vi "file read and write.vi"() -> (2 "data match?":bool)   [LabVIEW 2013, in "Shared Memory Tests.lvlib"]
uses:
  Shared Memory Tests.lvlib
  module/execution/Shared Memory Runtime.lvclass
  module/configuration/Shared Memory Configuration.lvclass
  <vilib>/NI/Tag Bus/dictionary/data dictionary.lvclass/data dictionary.ctl
  <vilib>/Analysis/1siggen.llb/Ramp Pattern by Samples.vi
  <vilib>/NI/Tag Bus/dictionary/lookup polymorphs/locate double.vi
  <vilib>/NI/Tag Bus/table/data polymorphs/write many/write Doubles.vi
  <vilib>/NI/Tag Bus/table/data polymorphs/read many/read Doubles.vi
  <vilib>/NI/Tag Bus/dictionary/search/find data index.vi
  <vilib>/NI/Tag Bus/dictionary/search/search string list.vi
  <vilib>/NI/Tag Bus/dictionary/tag not found.vi
  <vilib>/Analysis/NI_AALBase.lvlib
  <vilib>/NI/Tag Bus/table/data table.lvlib
  <vilib>/NI/Tag Bus/dictionary/data dictionary.lvclass
panel:
  out "error out":errorcluster
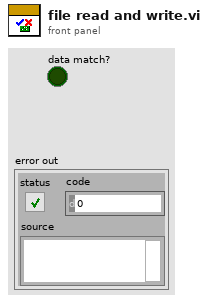
[diagram p1: front panel]
types:
  T1 = typedef "TBM channel.lvclass/data tables.ctl" = cluster{"input data":T2, "processing parameter":T2, "processing result":T2, "output data":T2}
  T2 = typedef "tag bus.lvlib/dictionary table pair.ctl" = cluster{"data dictionary":refnum<class "data dictionary.lvclass">, "data table":T3}
  T3 = typedef "tag bus.lvlib/data table.lvlib/data table.ctl" = cluster{"Double":dbl[], "Single":sgl[], "I64":i64[], "I32":i32[], "I16":i16[], "I8":i8[], "U64":u64[], "U32":u32[], "U16":u16[], "U8":u8[], "Boolean":bool[], "String":string[], "Array of Double":cluster{"DBL Array":dbl[]}[], "Array of Single":cluster{"SGL Array":sgl[]}[], "Array of I64":cluster{"I64 Array":i64[]}[], "Array of I32":cluster{"I32 Array":i32[]}[], "Array of I16":cluster{"I16 Array":i16[]}[], "Array of I8":cluster{"I8 Array":i8[]}[], "Array of U64":cluster{"U64 Array":u64[]}[], "Array of U32":cluster{"U32 Array":u32[]}[], "Array of U16":cluster{"U16 Array":u16[]}[], "Array of U8":cluster{"U8 Array":u8[]}[], "Array of Boolean":cluster{"Boolean Array":bool[]}[], "Array of String":cluster{"String Array":string[]}[]}
  T4 = typedef "tag bus.lvlib/data dictionary.lvclass/full data dictionary.ctl" = cluster{"Double":string[], "Single":string[], "I64":string[], "I32":string[], "I16":string[], "I8":string[], "U64":string[], "U32":string[], "U16":string[], "U8":string[], "Boolean":string[], "String":string[], "Array of Double":string[], "Array of Single":string[], "Array of I64":string[], "Array of I32":string[], "Array of I16":string[], "Array of I8":string[], "Array of U64":string[], "Array of U32":string[], "Array of U16":string[], "Array of U8":string[], "Array of Boolean":string[], "Array of String":string[]}
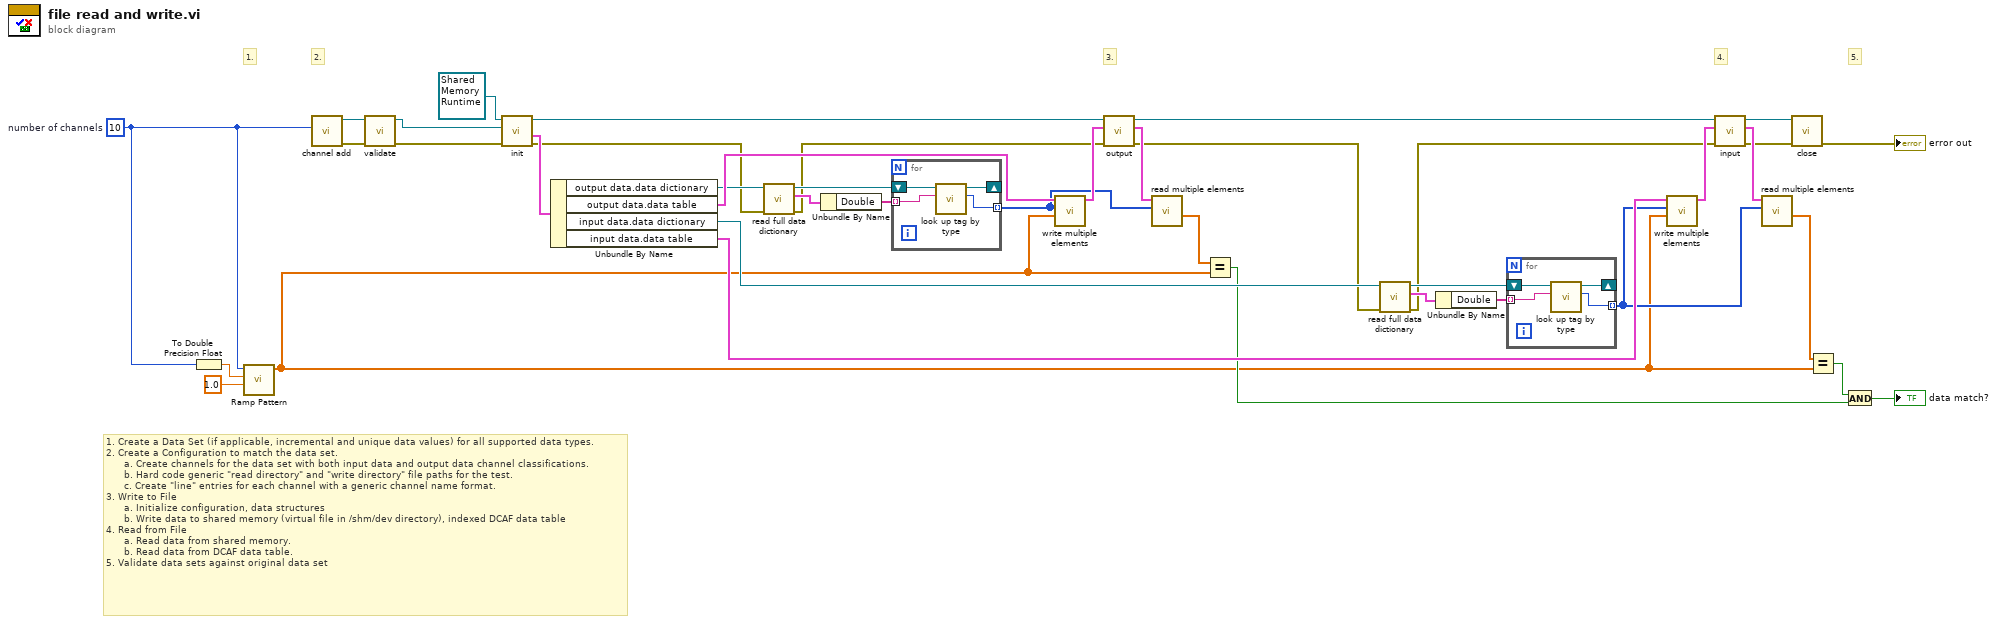
[diagram p0: block diagram]
diagram:
  w14 = 10  # number of channels
  # "5."
  # "4."
  # "3."
  # "2."
  # "1."
  # "1. Create a Data Set (if applicable, incremental and unique data values) for all supported data types.\n2. Create a Configuration to match the data set.\n      a. Create channels for the data set with both input data and output data channel classifications.\n      b. Hard code generic \"read directory\" and \"write directory\" file paths for the test.\n      c. Create \"line\" entries for each channel with a generic channel name format.\n3. Write to File\n      a. Initialize configuration, data structures\n      b. Write data to shared memory (virtual file in /shm/dev directory), indexed DCAF data table\n4. Read from File\n      a. Read data from shared memory.\n      b. Read data from DCAF data table.\n5. Validate data sets against original data set"
  n1 = To Double Precision Float(number=w14) -> (double precision float=w35:dbl)
  n2 = call-poly <vilib>:"Ramp Pattern.vi"("start"=1.0, "end"=w35, "samples"=w14) -> ("Ramp Pattern"=w1:dbl[])  [unwired: 7 in, 1 out]
  n3 = call "channel add.vi"("number of channels (1)"=w14) -> ("error out"=w33:errorcluster, "configuration out"=w32:refnum<class "Shared Memory Configuration.lvclass">)  [unwired: 6 in, 3 out]
  n4 = call-dynamic "validate.vi"("error in"=w33, "shared memory module configuration"=w32) -> ("error out"=w30:errorcluster, "shared memory module configuration out"=w31:refnum<class "Shared Memory Configuration.lvclass">)  [unwired: 8 in]
  n5 = call-dynamic "init.vi"("error in"=w30, "TBM module configuration in"=w31, "shared memory module runtime"=refnum<class "Shared Memory Runtime.lvclass"> refnum) -> ("error out"=w2:errorcluster, "data allocations"=w34:T1, "shared memory module runtime out"=w3:refnum<class "Shared Memory Runtime.lvclass">)  [unwired: 5 in, 1 out]
  n6 = Unbundle By Name(w34) -> ("output data.data dictionary"=w28:refnum<class "data dictionary.lvclass">, "output data.data table"=w29:T3, "input data.data dictionary"=w18:refnum<class "data dictionary.lvclass">, "input data.data table"=w15:T3)
  n7 = call <vilib>:"read full data dictionary.vi"("error in"=w2, "data dictionary in"=w28) -> ("error out"=w17:errorcluster, "dictionary"=w27:T4, "data dictionary out"=w26:refnum<class "data dictionary.lvclass">)  [unwired: 7 in]
  n8 = Unbundle By Name(w27) -> ("Double"=w25:string[])
  n9 = for {
    shift-right: [w43] -> _
    shift-left: w26 -> [w44]
    tunnel: w25 -> [w42] mode=indexing
    tunnel: [w41] -> w23 mode=indexing
    n10 = call-poly <vilib>:"look up tag by type.vi"("name"=w42, "data dictionary in"=w44) -> ("index"=w41:i32, "data dictionary out"=w43:refnum<class "data dictionary.lvclass">)  [unwired: 7 in, 1 out]
  }
  n11 = call-poly <vilib>:"write multiple elements.vi"("values"=w1, "indices"=w23, "data table in"=w29) -> ("data table out"=w39:T3)  [unwired: 8 in]
  n12 = call-dynamic "output.vi"("error in"=w17, "output data table"=w39, "shared memory module"=w3) -> ("error out"=w16:errorcluster, "output data table out"=w24:T3, "shared memory module out"=w8:refnum<class "Shared Memory Runtime.lvclass">)  [unwired: 6 in]
  n13 = call-poly <vilib>:"read multiple elements.vi"("indices"=w23, "data table in"=w24) -> ("values"=w22:dbl[])  [unwired: 8 in, 1 out]
  n14 = Equal?(x=w22, y=w1) -> (x = y?=w10:bool)
  n15 = call <vilib>:"read full data dictionary.vi"("error in"=w16, "data dictionary in"=w18) -> ("error out"=w7:errorcluster, "dictionary"=w19:T4, "data dictionary out"=w20:refnum<class "data dictionary.lvclass">)  [unwired: 7 in]
  n16 = Unbundle By Name(w19) -> ("Double"=w21:string[])
  n17 = for {
    shift-right: [w47] -> _
    shift-left: w20 -> [w48]
    tunnel: w21 -> [w46] mode=indexing
    tunnel: [w45] -> w12 mode=indexing
    n18 = call-poly <vilib>:"look up tag by type.vi"("name"=w46, "data dictionary in"=w48) -> ("index"=w45:i32, "data dictionary out"=w47:refnum<class "data dictionary.lvclass">)  [unwired: 7 in, 1 out]
  }
  n19 = call-poly <vilib>:"write multiple elements.vi"("values"=w1, "indices"=w12, "data table in"=w15) -> ("data table out"=w13:T3)  [unwired: 8 in]
  n20 = call-dynamic "input.vi"("error in"=w7, "input data table in"=w13, "shared memory module"=w8) -> ("error out"=w5:errorcluster, "input data table out"=w38:T3, "shared memory module out"=w6:refnum<class "Shared Memory Runtime.lvclass">)  [unwired: 6 in]
  n21 = call-poly <vilib>:"read multiple elements.vi"("indices"=w12, "data table in"=w38) -> ("values"=w37:dbl[])  [unwired: 8 in, 1 out]
  n22 = call-dynamic "close.vi"("error in"=w5, "shared memory module runtime"=w6) -> ("error out"=→"error out":errorcluster)  [unwired: 9 in]
  n23 = Equal?(x=w37, y=w1) -> (x = y?=w11:bool)
  n24 = And(x=w11, y=w10) -> (x .and. y?=→"data match?":bool)
